vi "ReserveRef.vi"(0 "DashboardServer in":refnum<class "Dashboard Server.lvclass">, 5 "error in (no error)":errorcluster) -> (14 "DashboardServer out":refnum<class "Dashboard Server.lvclass">, 19 "error out":errorcluster)   [LabVIEW 2016, in "Dashboard Server.lvclass"]
uses:
  Dashboard Server.lvclass
  Dashboard Server.lvclass/Dashboard Server.ctl
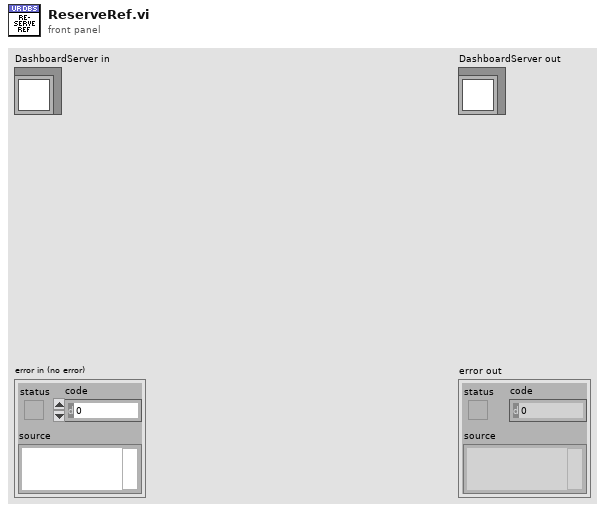
[diagram p1: front panel]
types:
  T1 = typedef "Semaphore RefNum" = refnum<k1>
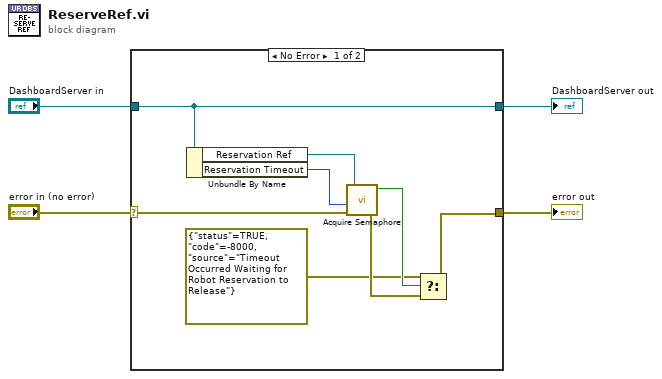
[diagram p0: block diagram]
diagram:
  n1 = case shown="No Error" "error in (no error)" {
    selector: "error in (no error)" -> [w11 w14]
    tunnel: [w6 w14] -> w3
    tunnel: [w12 w13] -> w1
    tunnel: "DashboardServer in" -> [w12 w13]
    frame No Error {
      n2 = Unbundle By Name(w12) -> ("Reservation Ref"=w10:T1, "Reservation Timeout"=w9:i32)
      n3 = call <vilib>:"Acquire Semaphore.vi"("error in (no error)"=w11, "ms timeout (-1)"=w9, "semaphore"=w10) -> ("error out"=w7:errorcluster, "timed out"=w8:bool)  [unwired: 2 in, 1 out]
      n4 = Select(t=errorcluster {"status"=TRUE, "code"=-8000, "source"="Timeout Occurred Waiting for Robot Reservation to Release"} ("error constant"), s=w8, f=w7) -> (s? t:f=w6:errorcluster)
    }
    frame Error {
    }
  }
  "error out" <- w3
  "DashboardServer out" <- w1
